vi "Autotuning PID Online and Inline.vi"() -> ()   [LabVIEW 2015]
doc: "This example demonstrates how to use the PID Online Autotuning VI with the PID algorithm in series with the VI."
uses:
  <vilib>/addons/control/pid/NI_PID_autopid.lvlib
  <vilib>/addons/control/pid/NI_PID_pid.lvlib
  <vilib>/addons/control/pid/pid.llb/PID Advanced (DBL).vi
  <vilib>/addons/control/pid/autopid.llb/PID Online Autotuning (Relay Feedback).vi
panel:
  in  "gamma":dbl(slide)=0.5102040816326531 scale=0.0..1.0
  out "tuning completed?":bool
  in  "Tab Control":enum32{"Instructions", "Plant Parameters"}(tab)
  in  "Instructions":string="Overview: This example demonstrates how to use the  PID Online Autotuning VI with the PID using the Relay Autotuning Technique.\nInstructions:\n1. Run the VI and wait until the process variable (PV) reaches near setpoint (SP).\n2.  On the PID Autotuning Design section, select the type of algorithm, type of controller and excitation amplitude for the 'open loop step response'. Then, click Autotune to start the process.\n3.  When the tuned PID gains do not change anymore or the tuning completed? flashes, the identification is done and you can accept new gains by pressing Accept gain and that will transfer the new gain to PID Gains.\n4. Click Autotune again to go back to the automatic control. You can try different options and repeat this process.\n5. Click Stop to stop the VI.\n"
  out "Plant Variable Gain":dbl=5.68817109595442
  out "Plant Variable Lag":dbl=1.4596237458843302
  in  "Load":dbl(slide) scale=0.0..10.0
  in  "alpha":dbl(slide)=0.49999999999999994 scale=0.0..1.0
  in  "Automatic":bool=TRUE
  in  "Reinitialize":bool
  in  "autotuning parameters":T1={"Type of Controller"=0, "relay cycles"=3, "relay amplitude"=1.0, "control specifications"=2, "PV noise level"=0.1} {"PV noise level" format="%.2f"; "control specifications" items=["fast", "normal", "slow"]; "relay amplitude" format="%.2f"; "Type of Controller" items=["P", "PI", "PID"]}
  out "MV":dbl(graph)=20.39115328927357
  in  "Accept gain":bool
  out "tuned PID gains":T2={"proportional gain (Kc)"=1.9838195929127882, "integral time (Ti, min)"=0.01995856284686879, "derivative time (Td, min)"=0.0} {"derivative time (Td, min)" format="%#.6g"; "integral time (Ti, min)" format="%#.6g"; "proportional gain (Kc)" format="%#.6g"}
  in  "Autotune":bool
  in  "SP:":dbl(slide)=28.758169934640524 min=0.0 max=0.0 scale=0.0..100.0
  in  "MV:":dbl(slide)=0.015865722743421174 scale=-100.0..100.0
  out "PV:":dbl(slide)=28.4408554797721 scale=0.0..100.0
  in  "PID Gains":T2={"proportional gain (Kc)"=0.05, "integral time (Ti, min)"=0.0, "derivative time (Td, min)"=0.0} {"derivative time (Td, min)" format="%#.6g"; "integral time (Ti, min)" format="%#.6g"; "proportional gain (Kc)" format="%#.6g"}
  in  "Sampling Time dt (s)":dbl=0.05 min=0.001 step=0.01 format="%#.3p"
  in  "Stop":bool
  out "SP and PV":cluster{"initial PV":dbl, "SP1:":dbl}(graph)={"initial PV"=50.98160323470328, "SP1:"=50.98039215686275}
  # "Proportional-Integral-Derivative (PID) Controller"
  # "PID Autotuning Design"
  # "Plant Simulated Parameters"
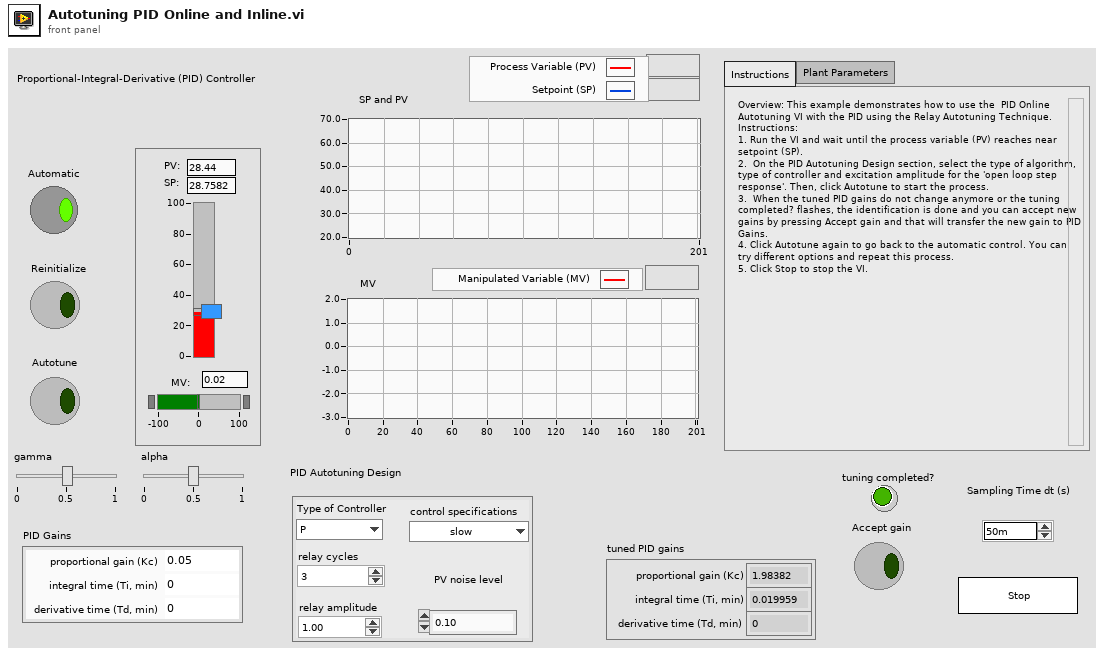
[diagram p1: front panel]
types:
  T1 = cluster{"Type of Controller":u16, "relay cycles":i32, "relay amplitude":dbl, "control specifications":u16, "PV noise level":dbl}
  T2 = cluster{"proportional gain (Kc)":dbl, "integral time (Ti, min)":dbl, "derivative time (Td, min)":dbl}
  T3 = cluster{"static gain":dbl, "lag (s)":dbl, "deadtime (s)":dbl, "load":dbl, "deadband":dbl, "sensor noise":dbl, "initial PV":dbl, "plant noise":dbl}
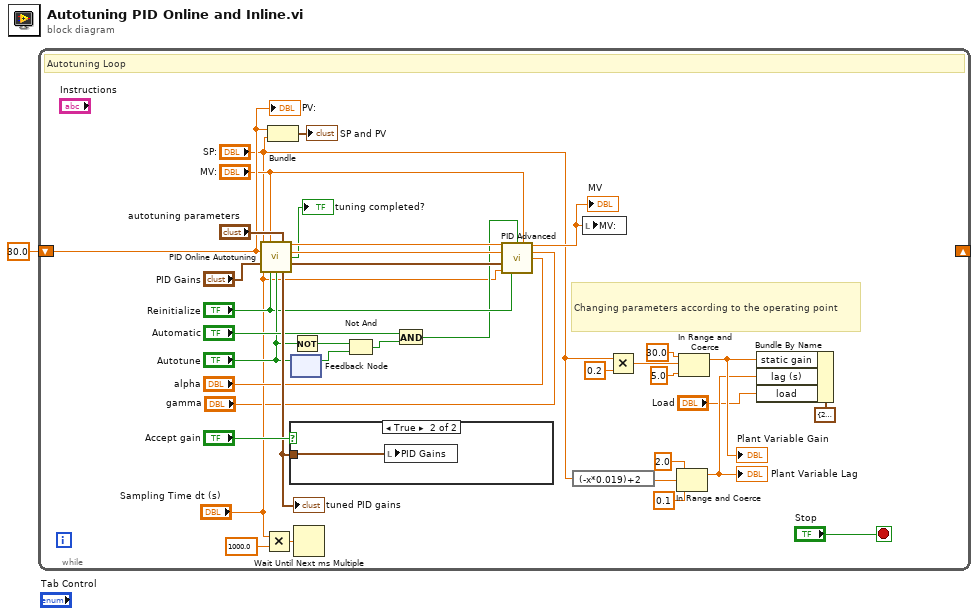
[diagram p0: block diagram]
diagram:
  n1 = while {
    shift-left: 30.0 -> [w21]
    shift-right: _ -> [_]
    stop <- "Stop" stop-if-true
    # "Changing parameters according to the operating point"
    # "Autotuning Loop"
    n2 = call-poly <vilib>:"PID Online Autotuning.VI"("setpoint"="SP:", "manipulated variable"="MV:", "autotuning parameters"="autotuning parameters", "process variable"=w21, "PID gains in"="PID Gains", "dt (s)"="Sampling Time dt (s)", "reinitialize? (F)"="Reinitialize", "autotune? (F)"="Autotune") -> ("setpoint out"=w28:dbl, "process variable out"=w27:dbl, "tuning completed?"=→"tuning completed?":bool, "PID gains out"=w23:T2, "tuned PID gains"=w22:T2)  [unwired: 3 in]
    "tuned PID gains" <- w22
    n3 = Multiply(x="Sampling Time dt (s)", y=1000.0) -> (x*y=w2:dbl)
    n4 = Bundle(w21, "SP:"="SP:") -> (→"SP and PV":cluster{dbl, "SP:":dbl})  [unwired: 1 in]
    n5 = case shown="True" "Accept gain" {
      tunnel: w22 -> [_ w39]
      frame False {
      }
      frame True {
        n6 = local write "PID Gains"(w39) -> ()
      }
    }
    n7 = feedback #1() -> (w17:bool)  [unwired: 1 in]
    n8 = feedback-in #1("Autotune") -> ()
    n9 = Not(x="Autotune") -> (.not. x?=w14:bool)
    n10 = Wait Until Next ms Multiple(millisecond multiple=w2) -> ()  [unwired: 1 out]
    n11 = Not And(1:w17, 2:w14) -> (0:w15:bool)
    n12 = And(x="Automatic", y=w15) -> (x .and. y?=w5:bool)
    n13 = call-poly <vilib>:"PID Advanced.vi"("setpoint"=w28, "auto? (T)"=w5, "manual control"="MV:", "process variable"=w27, "gamma"="gamma", "alpha"="alpha", "PID gains"=w23, "dt (s)"="Sampling Time dt (s)", "reinitialize? (F)"="Reinitialize") -> ("output"=w20:dbl)  [unwired: 5 in, 1 out]
    "MV" <- w20
    n14 = expression code="(-x*0.019)+2"("SP:") -> (w29:dbl)
    n15 = local write "MV:"(w20) -> ()
    n16 = Multiply(x="SP:", y=0.2) -> (x*y=w33:dbl)
    n17 = In Range and Coerce(upper limit=2.0, x=w29, lower limit=0.1) -> (coerced(x)=w10:dbl)  [unwired: 1 out]
    "Plant Variable Lag" <- w10
    n18 = In Range and Coerce(upper limit=30.0, x=w33, lower limit=5.0) -> (coerced(x)=w11:dbl)  [unwired: 1 out]
    "Plant Variable Gain" <- w11
    n19 = Bundle By Name(cluster=T3 {"static gain"=2.5, "lag (s)"=2.5, "deadtime (s)"=0.5, "load"=0.0, "deadband"=0.0, "sensor noise"=0.0, "initial PV"=30.0, "plant noise"=0.0} ("process parameters"), "static gain"=w11, "lag (s)"=w10, "load"="Load") -> ()  [unwired: 1 out]
    "PV:" <- w21
  }
